vi "LS330_ArrayClear.vi"(9 "Clear":bool, 10 "input cluster":T1) -> (2 "output cluster":T1)   [LabVIEW 2021]
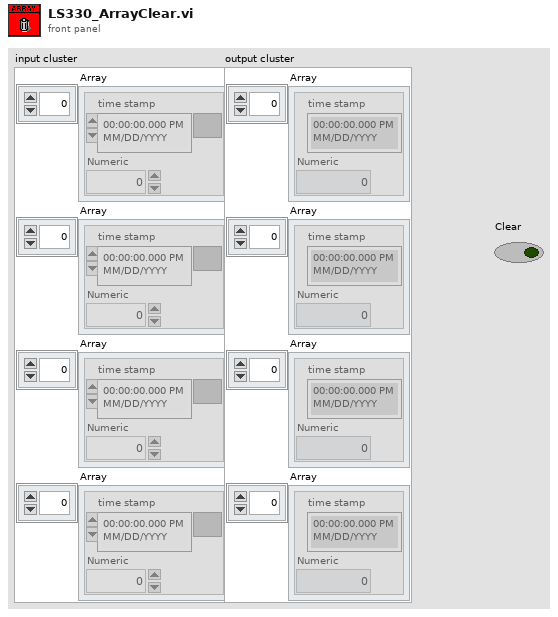
[diagram p1: front panel]
types:
  T1 = cluster{"Array":cluster{"time stamp":timestamp, "Numeric":dbl}[], "Array":cluster{"time stamp":timestamp, "Numeric":dbl}[], "Array":cluster{"time stamp":timestamp, "Numeric":dbl}[], "Array":cluster{"time stamp":timestamp, "Numeric":dbl}[]}
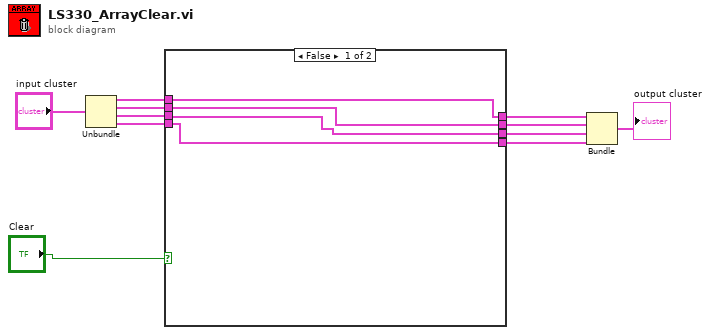
[diagram p0: block diagram]
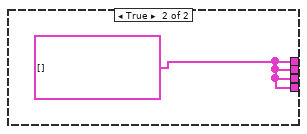
[diagram p2: hidden frame]
diagram:
  n1 = Unbundle("input cluster") -> ("Array"=w9:cluster{"time stamp":timestamp, "Numeric":dbl}[], "Array"=w8:cluster{"time stamp":timestamp, "Numeric":dbl}[], "Array"=w7:cluster{"time stamp":timestamp, "Numeric":dbl}[], "Array"=w6:cluster{"time stamp":timestamp, "Numeric":dbl}[])
  n2 = case shown="False" "Clear" {
    tunnel: w9 -> [w15 _]
    tunnel: w8 -> [w14 _]
    tunnel: w7 -> [w13 _]
    tunnel: w6 -> [w12 _]
    tunnel: [w15 w16] -> w4
    tunnel: [w14 w16] -> w2
    tunnel: [w13 w16] -> w3
    tunnel: [w12 w16] -> w1
    frame False {
    }
    frame True {
      w16 = cluster{"time stamp":timestamp, "Numeric":dbl}[] [] ("Array")
    }
  }
  n3 = Bundle("Array"=w4, "Array"=w2, "Array"=w3, "Array"=w1) -> (→"output cluster":T1)  [unwired: 1 in]
